vi "Exit Windows.vi"(6 "show prompt? (T)":bool=TRUE, 7 "退出Windows函数 (1)":T1(ring)=enum."Shut Down") -> ()   [LabVIEW 2011, in "API.lvlib"]
doc: "This VI allows you to exit windows in various ways.\nexit windows function\n0: Log off\n1: Shut Down\n2: Exit Windows and reboot the computer"
uses:
  API.lvlib
  user32.dll
panel:
  out "error out":errorcluster caption="错误输出"
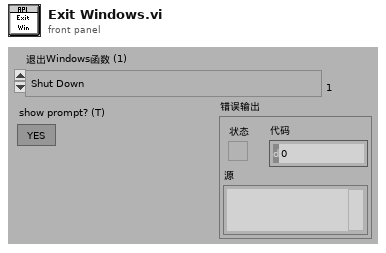
[diagram p1: front panel]
types:
  T1 = enum16{"Log off", "Shut Down", "Exit Windows and Reboot"}
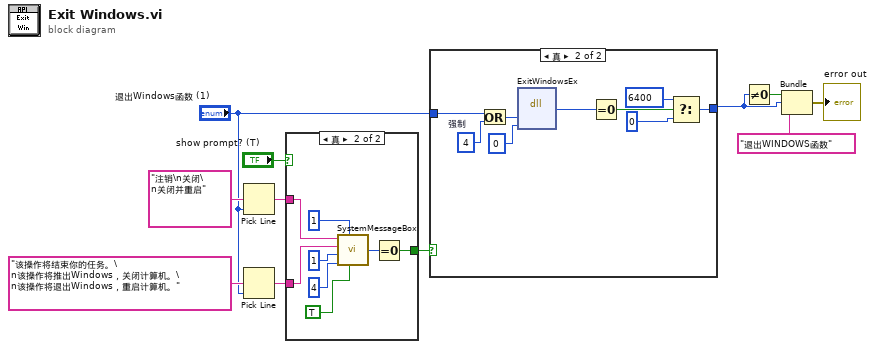
[diagram p0: block diagram]
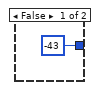
[diagram p2: hidden frame]
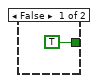
[diagram p3: hidden frame]
diagram:
  n1 = Pick Line(multi-line string="注销\n关闭\n关闭并重启", line index="退出Windows函数 (1)") -> (output string=w7:string)  [unwired: 1 in]
  n2 = Pick Line(multi-line string="该操作将结束你的任务。\n该操作将推出Windows，关闭计算机。\n该操作将退出Windows，重启计算机。", line index="退出Windows函数 (1)") -> (output string=w6:string)  [unwired: 1 in]
  n3 = case shown="真" "show prompt? (T)" {
    tunnel: [TRUE w19] -> w10
    tunnel: w7 -> [_ w14]
    tunnel: w6 -> [_ w13]
    frame False {
    }
    frame True {
      n4 = call "SystemMessageBox.vi"("sound? (F)"=TRUE, "modality (0)"=1, "icon (0:None)"=4, "buttons (0:OK)"=1, "message (\"\")"=w13, "window title (\"\")"=w14) -> ("button pressed"=w18:i32)
      n5 = Equal To 0?(x=w18) -> (x = 0?=w19:bool)
    }
  }
  n6 = case shown="真" w10 {
    tunnel: [-43 w30] -> w4
    tunnel: "退出Windows函数 (1)" -> [_ w24]
    frame False {
    }
    frame True {
      w23 = u32 4  # 强制
      n7 = Or(x=w24, y=w23) -> (x .or. y?=w22:u32)
      n8 = dll-call lib="user32.dll" fn="ExitWindowsEx" label="ExitWindows"("returnCode"=w22, "reserved (set to zero)"=u32 0) -> ("返回类型"=w26:i32)  [unwired: 5 in, 2 out]
      n9 = Equal To 0?(x=w26) -> (x = 0?=w27:bool)
      n10 = Select(t=6400, s=w27, f=0) -> (s? t:f=w30:i32)
    }
  }
  n11 = Not Equal To 0?(x=w4) -> (x != 0?=w5:bool)
  n12 = Bundle(w5, w4, "退出WINDOWS函数") -> (→"error out":errorcluster)  [unwired: 1 in]
